vi "Test API Execution from Class object Returns Method Results.vi"(8 "error in (no error)":errorcluster, 11 "API Test in":refnum<class "API Test.lvclass">) -> (0 "error out":errorcluster, 3 "API Test out":refnum<class "API Test.lvclass">)   [LabVIEW 2020, in "LUnit Tests.lvlib" / "API Test.lvclass"]
uses:
  API Test.lvclass
  C:/Program Files (x86)/National Instruments/LabVIEW 2020/vi.lib/Asteme/LUnit/Test Case.lvclass
  Test Dummys/Test Test Case/Test Test Case.lvclass
  C:/Users/anton/Documents/GitHub/LUnit/source/Framework/Test Case/LUnit Test Case.lvclass
  <vilib>/Asteme/LUnit/Test Case.lvclass/Test Case.ctl
  <vilib>/Asteme/LUnit/LUnit Assertion Result.lvclass/LUnit Assertion Result.ctl
  <vilib>/Asteme/LUnit/LUnit Test Case Result.lvclass/LUnit Test Case Result.ctl
  <vilib>/Asteme/LUnit/LUnit Method Result.lvclass/LUnit Method Result.ctl
  <vilib>/Asteme/LUnit/Palette/Fail.vi
  <vilib>/Asteme/LUnit/Palette/Pass.vi
  <vilib>/Asteme/LUnit/Set Assertion Type.vi
  <vilib>/Asteme/LUnit/Add test result.vi
  <vilib>/Asteme/LUnit/LUnit Write Passed.vi
  <vilib>/Asteme/LUnit/LUnit Write Message.vi
  <vilib>/Asteme/LUnit/LUnit Write Description.vi
  <vilib>/Asteme/LUnit/LUnit Write Assertion Type.vi
  <vilib>/Asteme/LUnit/LUnit Record Assertion Result.vi
  <vilib>/Asteme/LUnit/LUnit Aggregate Assertion Results.vi
  <vilib>/Asteme/LUnit/Assertion Result/LUnit Read Status.vi
  <vilib>/Asteme/LUnit/LUnit Read Message.vi
  <vilib>/Asteme/LUnit/LUnit Read Description.vi
  <vilib>/Asteme/LUnit/Method Result/LUnit Merge Status.vi
  <vilib>/Asteme/LUnit/LUnit Concatenate result strings.vi
  <vilib>/Asteme/LUnit/LUnit Assertion Result.lvclass
  source/Framework/Execution API/Execution API.lvclass
  <vilib>/Asteme/LUnit/Test Case.lvclass
  C:/Users/anton/Documents/GitHub/LUnit/tests/Test Dummys/Test Test Case/Test Test Case.lvclass
  C:/Users/anton/Documents/GitHub/LUnit/tests/API Test/API Test.lvclass
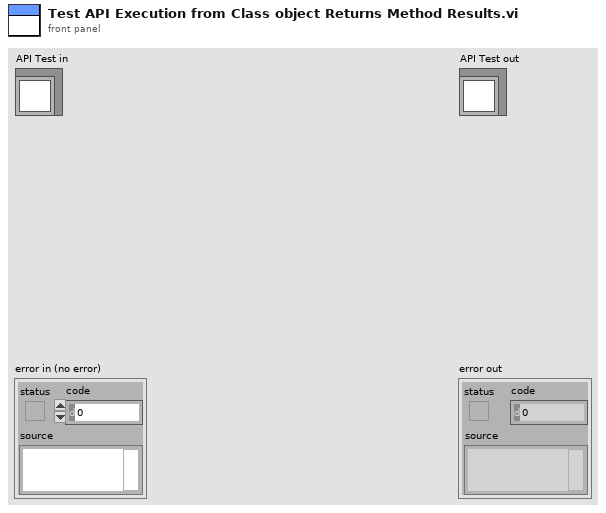
[diagram p1: front panel]
types:
  T1 = cluster{"Event Registration Refnum":refnum<event-registration>, "Event Registration Refnum":refnum<event-registration>}
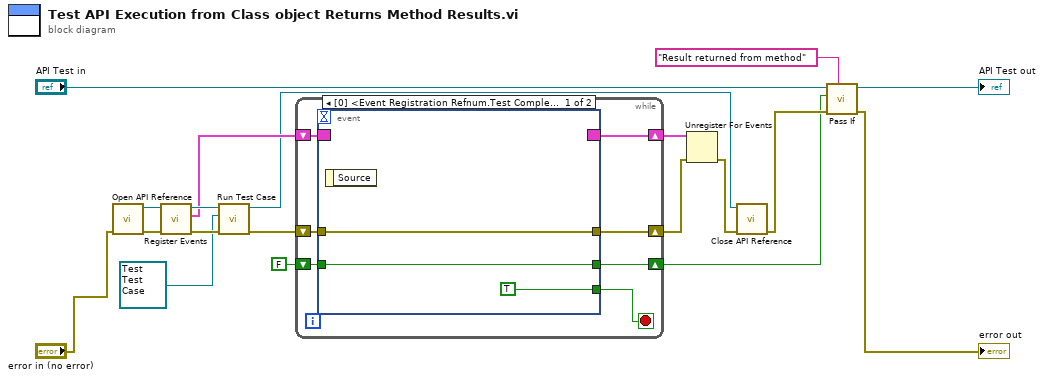
[diagram p0: block diagram]
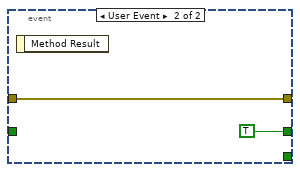
[diagram p2: hidden frame]
diagram:
  n1 = call "Open API Reference.vi"("error in (no error)"="error in (no error)") -> ("error out"=w18:errorcluster, "Execution API out"=w19:refnum<class "Execution API.lvclass">)  [unwired: 9 in]
  n2 = call "Register Events.vi"("error in (no error)"=w18, "Execution API In"=w19) -> ("error out"=w16:errorcluster, "Result Events"=w15:T1, "Execution API Out"=w17:refnum<class "Execution API.lvclass">)  [unwired: 7 in]
  n3 = call "Run Test Case.vi"("error in (no error)"=w16, "Test Case"=refnum<class "Test Test Case.lvclass"> refnum ("Framework Tests.lvlib:Test Test Case.lvclass"), "Execution API In"=w17) -> ("error out"=w12:errorcluster, "Execution API Out"=w8:refnum<class "Execution API.lvclass">)  [unwired: 7 in]
  n4 = while {
    shift-right: [w25] -> w14
    shift-left: w15 -> [w26]
    shift-right: [w23] -> w11
    shift-left: w12 -> [w24]
    shift-right: [w21] -> w2
    shift-left: FALSE -> [w20]
    stop <- w22 stop-if-true
    n5 = event shown="[0] <Event Registration Refnum.Test Completed>: User Event" {
      selector: w26 -> [_ _]
      dyn-events: [_ _] -> w25
      timeout: _ -> [_ _]
      tunnel: w24 -> [w29 w31]
      tunnel: [w29 w31] -> w23
      tunnel: [TRUE _] -> w22
      tunnel: [w27 TRUE] -> w21
      tunnel: w20 -> [w27 _]
      event User Event {
        n6 = event-data() -> ()  [unwired: 1 in, 1 out]
      }
      event User Event {
        n7 = event-data() -> ()  [unwired: 1 in, 1 out]
      }
    }
  }
  n8 = Unregister For Events(event registration refnum=w14, error in=w11) -> (error out=w10:errorcluster)
  n9 = call "Close API Reference.vi"("error in (no error)"=w10, "Execution API in"=w8) -> ("error out"=w9:errorcluster)  [unwired: 9 in]
  n10 = call <vilib>:"Pass If.vi"("Description"="Result returned from method", "error in (no error)"=w9, "Pass?"=w2, "LUnit Test Case In"="API Test in") -> ("error out"=→"error out":errorcluster, "LUnit Test Case Out"=→"API Test out":refnum<class "API Test.lvclass">)  [unwired: 6 in]
